vi "Forward Data.vi"(8 "error in (no error)":errorcluster, 9 "Data":variant, 10 "Forwarding Case":T1, 11 "TCP Read in":refnum<class "DS TCP Read.lvclass">) -> (0 "error out":errorcluster, 3 "TCP Read out":refnum<class "DS TCP Read.lvclass">)   [LabVIEW 2017, in "DS TCP Server.lvlib" / "DS TCP Read.lvclass"]
uses:
  DS TCP Read.lvclass
  C:/Program Files (x86)/National Instruments/LabVIEW 2017/vi.lib/addons/_Workers/Library/Classes/Worker/Worker.lvclass
  <vilib>/addons/_Workers/Library/Case Label.ctl
  DS TCP Read.lvclass/DS TCP Read.ctl
  <vilib>/addons/_Workers/Library/Classes/Message/Priority (ALL).ctl
  <vilib>/addons/_Workers/Library/Classes/Worker/Worker.lvclass/Worker.ctl
  <vilib>/addons/_Workers/Library/Classes/Message/Message.lvclass/Message.ctl
  <vilib>/addons/_Workers/Library/Classes/Message Queue/Message Queue.lvclass/Message Queue.ctl
  <vilib>/addons/_Workers/Library/Classes/Message/Write Priority.vi
  <vilib>/addons/_Workers/Library/Classes/Message/Write Send Message to Debugger.vi
  <vilib>/addons/_Workers/Library/Classes/Message Queue/Enqueue Element.vi
  <vilib>/addons/_Workers/Library/Classes/Message/Write Time Stamp.vi
  <vilib>/addons/_Workers/Library/Classes/Message/Write Sender WID.vi
  <vilib>/addons/_Workers/Library/Classes/Message/Write Data.vi
  <vilib>/addons/_Workers/Library/Classes/Message/Write Recipient Case.vi
  <vilib>/addons/_Workers/Library/Classes/Message/Message Time Stamp.vi
  <vilib>/addons/_Workers/Library/Classes/Message/Write Sender Case.vi
  <vilib>/addons/_Workers/Library/Classes/Worker/Read Message.vi
  <vilib>/addons/_Workers/Library/Classes/Message/Read Recipient Case.vi
  <vilib>/addons/_Workers/Library/Classes/Message/Write Auxiliary.vi
  <vilib>/Utility/High Resolution Relative Seconds.vi
  <vilib>/Utility/error.llb/Error Cluster From Error Code.vi
  <vilib>/ErrorRing/Error Ring.xnode
  <vilib>/addons/_Workers/Library/Classes/Message/Message.lvclass
  <vilib>/addons/_Workers/Library/Classes/Message Queue/Message Queue.lvclass
  <vilib>/addons/_Workers/Library/Workers.lvlib
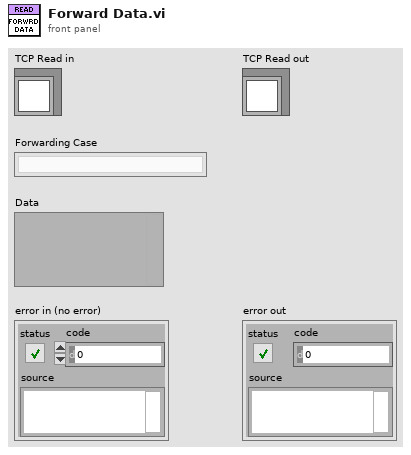
[diagram p1: front panel]
types:
  T1 = typedef "Workers.lvlib/Case Label.ctl" = string
  T2 = typedef "Workers.lvlib/Message.lvclass/Priority (ALL).ctl" = enum16{"Low", "Normal", "High", "Critical"}
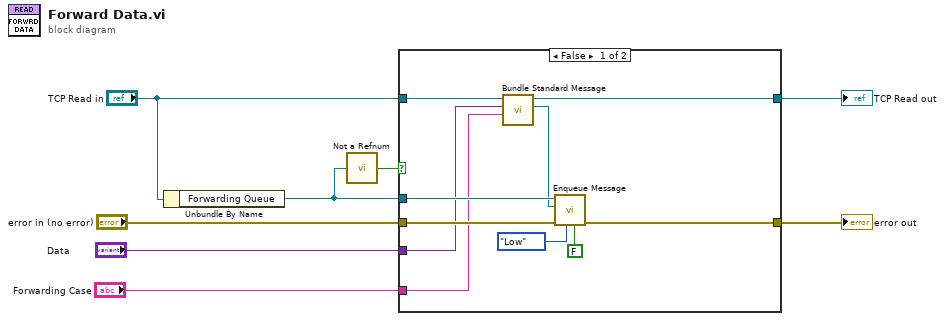
[diagram p0: block diagram]
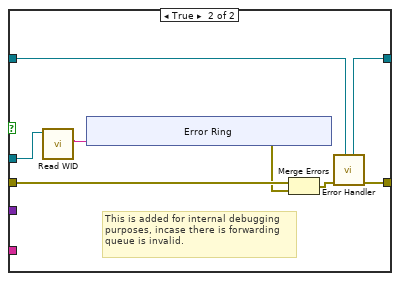
[diagram p2: hidden frame]
diagram:
  n1 = Unbundle By Name("TCP Read in") -> ("Forwarding Queue"=w4:refnum<class "Message Queue.lvclass">)
  n2 = call <vilib>:"Not a Refnum.vi"("Message Queue"=w4) -> ("Not a Refnum?"=w3:bool)  [unwired: 8 in]
  n3 = case shown="False" w3 {
    tunnel: "Data" -> [w12 _]
    tunnel: "Forwarding Case" -> [w11 _]
    tunnel: w4 -> [w16 w20]
    tunnel: "TCP Read in" -> [w15 w26]
    tunnel: [w14 w25] -> w7
    tunnel: [w17 w23] -> w6
    tunnel: "error in (no error)" -> [w18 w24]
    frame False {
      n4 = call <vilib>:"Bundle Standard Message.vi"("Case"=w11, "Data"=w12, "Worker"=w15) -> ("Message out"=w13:refnum<class "Message.lvclass">, "dup Worker out"=w14:refnum<class "DS TCP Read.lvclass">)  [unwired: 7 in]
      n5 = call <vilib>:"Enqueue Message.vi"("Send Message to Debugger? (T)"=FALSE, "Priority (Normal)"=Priority_(ALL)."Low", "error in"=w18, "Message"=w13, "Message Queue"=w16) -> ("error out"=w17:errorcluster)  [unwired: 6 in]
    }
    frame True {
      # "This is added for internal debugging\npurposes, incase there is forwarding\nqueue is invalid."
      n6 = call <vilib>:"Read WID.vi"("Message Queue in"=w20) -> ("WID"=w19:string)  [unwired: 9 in, 1 out]
      n7 = xnode "Error Ring"("parameter 0"=w19) -> ("error out"=w21:errorcluster)
      n8 = Merge Errors(w24, w21) -> (w22:errorcluster)
      n9 = call-dynamic "Error Handler.vi"("Worker"=w26, "error_in"=w22) -> ("error out"=w23:errorcluster, "Worker out"=w25:refnum<class "DS TCP Read.lvclass">)  [unwired: 7 in, 1 out]
    }
  }
  "TCP Read out" <- w7
  "error out" <- w6
